vi "trim_all_whitespace.vi"(10 "String":string) -> (2 "Trimmed String":string)   [LabVIEW 2020]
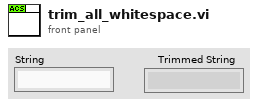
[diagram p1: front panel]
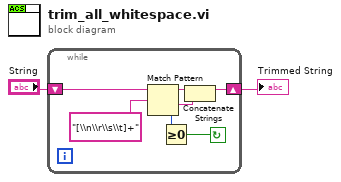
[diagram p0: block diagram]
diagram:
  n1 = while {
    shift-right: [w4] -> w1
    shift-left: "String" -> [w9]
    stop <- w7 continue-if-true
    n2 = Match Pattern(string=w9, regular expression="[\\n\\r\\s\\t]+") -> (before substring=w6:string, after substring=w5:string, offset past match=w8:i32)  [unwired: 2 out]
    n3 = Greater Or Equal To 0?(x=w8) -> (x >= 0?=w7:bool)
    n4 = Concatenate Strings(w6, w5) -> (w4:string)
  }
  "Trimmed String" <- w1
